vi "电压读取.vi"(4 "热电偶通道":string, 6 "NTC电阻":string, 8 "error in (no error)":errorcluster, 9 "实际电流":string, 10 "电压通道":string, 11 "VISA resource name":refnum<visa-resource-name>) -> (0 "error out":errorcluster, 3 "VISA resource name out":refnum<visa-resource-name>)   [LabVIEW 2021]
uses:
  <instrlib>/Keithley DMM6500 DAQ6500 Series/Public/Configure/Configure Temperature (Thermocouple).vi
  <instrlib>/Keithley DMM6500 DAQ6500 Series/Keithley DMM6500 DAQ6500 Series.lvlib
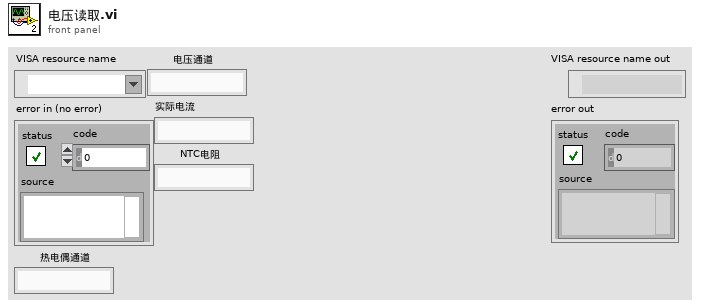
[diagram p1: front panel]
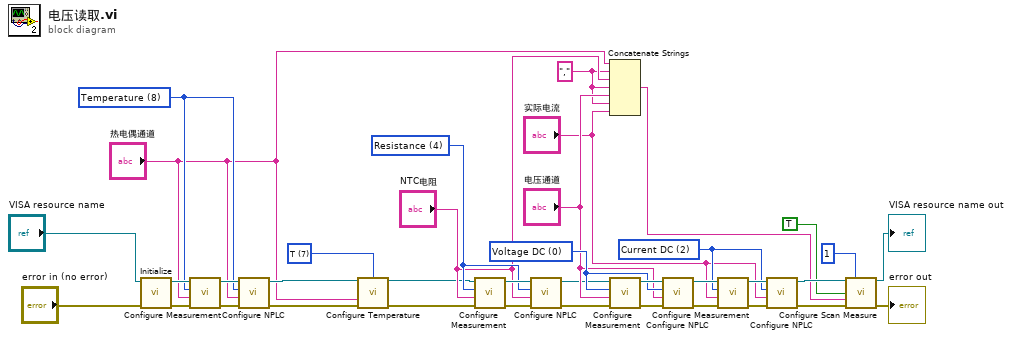
[diagram p0: block diagram]
diagram:
  w1 = 7 items=["B", "E", "J", "K", "N", "R", "S", "T"] ("Thermocouple Type (3: K)")
  w7 = 8 items=["Voltage DC", "Voltage AC", "Current DC", "Current AC", "Resistance", "4-wire Resistance", "Diode", "Capacitance", "Temperature", "Continuity", "Frequency", "Period", "Voltage Ratio", "Voltage", "Current"] ("Function (0: Voltage DC)")
  w14 = 4 items=["Voltage DC", "Voltage AC", "Current DC", "Current AC", "Resistance", "4-wire Resistance", "Diode", "Capacitance", "Temperature", "Continuity", "Frequency", "Period", "Voltage Ratio", "Voltage", "Current"] ("Function (0: Voltage DC)")
  w12 = "," ("字符串")
  w28 = 2 items=["Voltage DC", "Voltage AC", "Current DC", "Current AC", "Resistance", "4-wire Resistance", "Diode", "Capacitance", "Temperature", "Continuity", "Frequency", "Period", "Voltage Ratio", "Voltage", "Current"] ("Function (0: Voltage DC)")
  w33 = 0 items=["Voltage DC", "Voltage AC", "Current DC", "Current AC", "Resistance", "4-wire Resistance", "Diode", "Capacitance", "Temperature", "Continuity", "Frequency", "Period", "Voltage Ratio", "Voltage", "Current"] ("Function (0: Voltage DC)")
  n1 = call <instrlib>:"Initialize.vi"("error in (no error)"="error in (no error)", "VISA resource name"="VISA resource name") -> ("error out"=w10:errorcluster, "VISA resource name out"=w9:refnum<visa-resource-name>)  [unwired: 8 in]
  n2 = call <instrlib>:"Configure Measurement.vi"("error in (no error)"=w10, "Channel List(\"\")"="热电偶通道", "Function (0: Voltage DC)"=w7, "VISA resource name"=w9) -> ("error out"=w11:errorcluster, "VISA resource name out"=w8:refnum<visa-resource-name>)  [unwired: 6 in]
  n3 = call <instrlib>:"Configure NPLC.vi"("error in (no error)"=w11, "Channel List(\"\")"="热电偶通道", "Function (0: Voltage DC)"=w7, "VISA resource name"=w8) -> ("error out"=w6:errorcluster, "VISA resource name out"=w4:refnum<visa-resource-name>)  [unwired: 6 in]
  n4 = call-poly <instrlib>:"Configure Temperature.vi"("VISA resource name"=w4, "Thermocouple Type (3: K)"=w1, "Channel List(\"\")"="热电偶通道", "error in (no error)"=w6) -> ("VISA resource name out"=w3:refnum<visa-resource-name>, "error out"=w5:errorcluster)  [unwired: 10 in]
  n5 = call <instrlib>:"Configure Measurement.vi"("error in (no error)"=w5, "Channel List(\"\")"="NTC电阻", "Function (0: Voltage DC)"=w14, "VISA resource name"=w3) -> ("error out"=w18:errorcluster, "VISA resource name out"=w16:refnum<visa-resource-name>)  [unwired: 6 in]
  n6 = call <instrlib>:"Configure NPLC.vi"("error in (no error)"=w18, "Channel List(\"\")"="NTC电阻", "Function (0: Voltage DC)"=w14, "VISA resource name"=w16) -> ("error out"=w17:errorcluster, "VISA resource name out"=w15:refnum<visa-resource-name>)  [unwired: 6 in]
  n7 = Concatenate Strings("热电偶通道", w12, "NTC电阻", w12, "电压通道", w12, "实际电流") -> (w20:string)
  n8 = call <instrlib>:"Configure Measurement.vi"("error in (no error)"=w17, "Channel List(\"\")"="电压通道", "Function (0: Voltage DC)"=w33, "VISA resource name"=w15) -> ("error out"=w35:errorcluster, "VISA resource name out"=w34:refnum<visa-resource-name>)  [unwired: 6 in]
  n9 = call <instrlib>:"Configure NPLC.vi"("error in (no error)"=w35, "Channel List(\"\")"="电压通道", "Function (0: Voltage DC)"=w33, "VISA resource name"=w34) -> ("error out"=w29:errorcluster, "VISA resource name out"=w30:refnum<visa-resource-name>)  [unwired: 6 in]
  n10 = call <instrlib>:"Configure Measurement.vi"("error in (no error)"=w29, "Channel List(\"\")"="实际电流", "Function (0: Voltage DC)"=w28, "VISA resource name"=w30) -> ("error out"=w32:errorcluster, "VISA resource name out"=w31:refnum<visa-resource-name>)  [unwired: 6 in]
  n11 = call <instrlib>:"Configure NPLC.vi"("error in (no error)"=w32, "Channel List(\"\")"="实际电流", "Function (0: Voltage DC)"=w28, "VISA resource name"=w31) -> ("error out"=w25:errorcluster, "VISA resource name out"=w27:refnum<visa-resource-name>)  [unwired: 6 in]
  n12 = call <instrlib>:"Configure Scan Measure.vi"("VISA resource name"=w27, "Scan Count (0)"=u32 1, "Enable Scan Reset (T: Enable)"=TRUE, "Channel List(\"\")"=w20, "error in (no error)"=w25) -> ("VISA resource name out"=→"VISA resource name out":refnum<visa-resource-name>, "error out"=→"error out":errorcluster)  [unwired: 9 in]
